vi "decoupling_global.vi"() -> ()   [LabVIEW 2013]
uses:
  <vilib>/Analysis/Matrix/Datatypes/RealMatrix.ctl
  <vilib>/Analysis/Matrix/NI_Matrix.lvlib
panel:
  in  "Diff only":bool
  in  "Enable":bool
  in  "Decoupling matrix":T1=[[0.9965818996173275, 0.07528111013630094, -0.08121083864276656, -0.027893705147678832, 0.028105356058658888, -0.047018935935728284], [0.05396958333453812, 0.9938808243932792, -0.03250857338784263, -0.055876990314628915, -0.01603331171100984, -0.021224677010601753], [0.019895640482533002, 0.1795164361034258, 0.9924531316893929, 0.007229001103021841, -0.08565997961712835, 0.011213559362701209], [0.08712025868639314, 0.055860051656814985, -0.04184179527225186, 0.997195010064689, -0.004299202269350342, -0.041184891920432086], [0.01472712045877342, 0.07935288887894396, 0.000700308879555423, -0.05160338147098375, 0.9943011451805681, -0.07319095575228152], [0.11416364778116533, 0.031218189457441654, -0.014497547101663354, -0.07728505351149745, 0.06933689815823098, 0.991912602928943]] format="%#.3g"
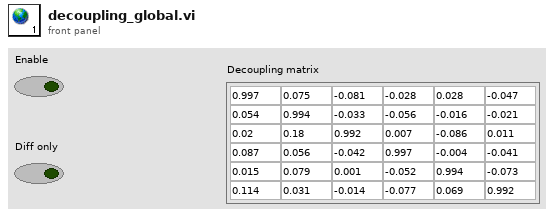
[diagram p1: front panel]
types:
  T1 = typedef "NI_Matrix.lvlib/RealMatrix.ctl" = dbl[][]
diagram:
